vi "Launcher.vi"() -> ()   [LabVIEW 2024]
uses:
  <vilib>/Utility/miscctls.llb/LVRectTypeDef.ctl
  Factory Folder/EngineFactory/EngineFactory.lvclass
  Client Folder/Client/Client.lvclass
  Product Folder/IMotor/IMotor.lvclass
  Product Folder/IECU/IECU.lvclass
  <vilib>/addons/GOOPUtility/GOOPUtility.lvlib
panel:
  out "Error Out":errorcluster
  out "Throttle Result":string
  out "Degree Result":string
  in  "Apply Throttle":bool
  in  "Apply Degree":bool
  in  "Throttle":dbl min=0.0 max=100.0 format="%#_g %"
  in  "Degree":dbl
  out "ECU Type":string
  out "Motor Type":string
  in  "Create Engine Button":bool
  in  "Engine Type":string(combo)
  # "ENGINE TYPE"
  # "ECU TYPE"
  # "MOTOR TYPE"
  # "DEGREE"
  # "THROTTLE"
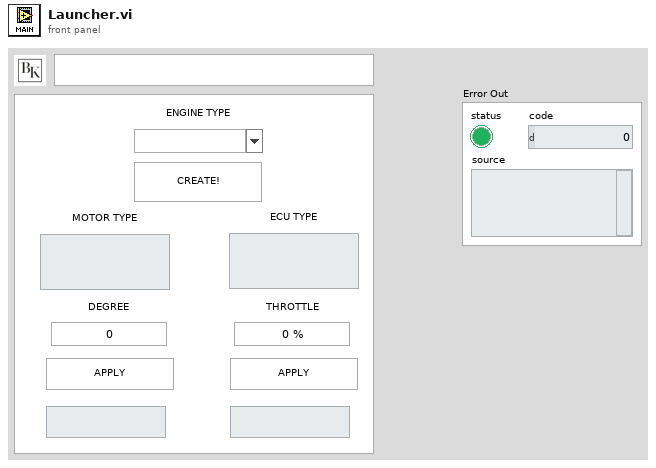
[diagram p1: front panel]
types:
  T1 = typedef "LVRectTypeDef.ctl" = cluster{"Left":i16, "Top":i16, "Right":i16, "Bottom":i16}
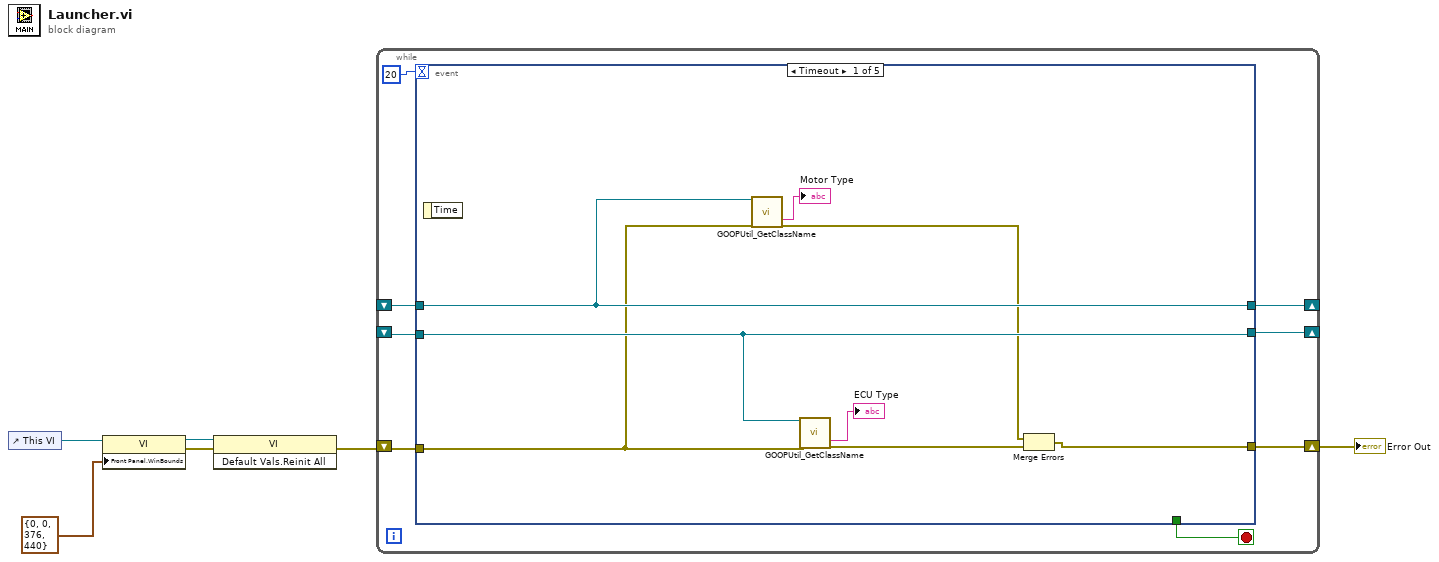
[diagram p0: block diagram]
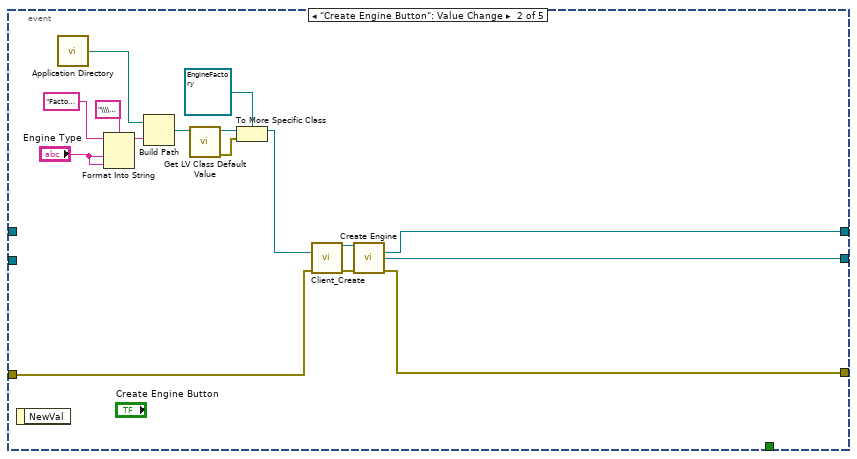
[diagram p2: hidden frame]
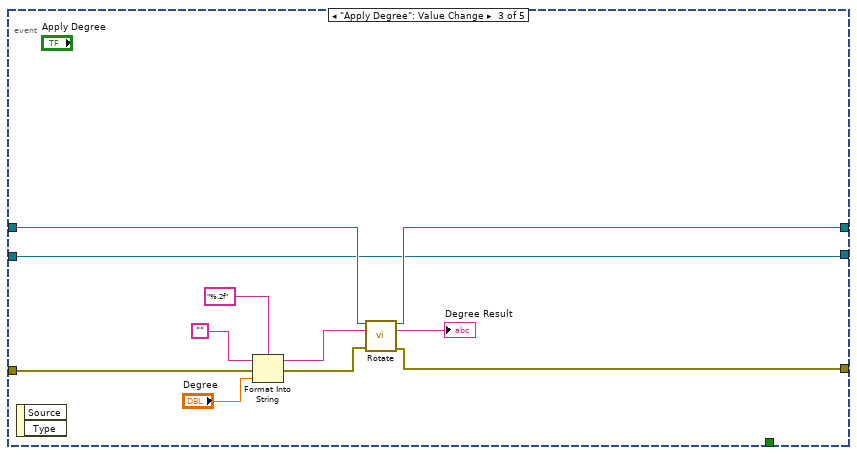
[diagram p3: hidden frame]
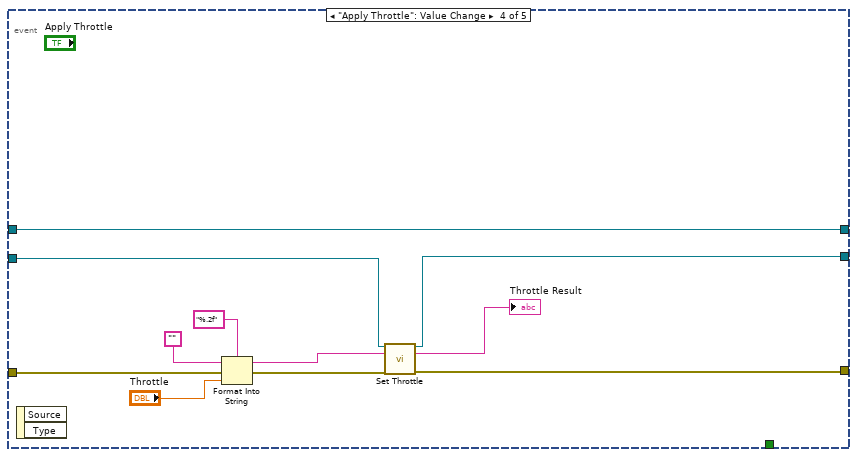
[diagram p4: hidden frame]
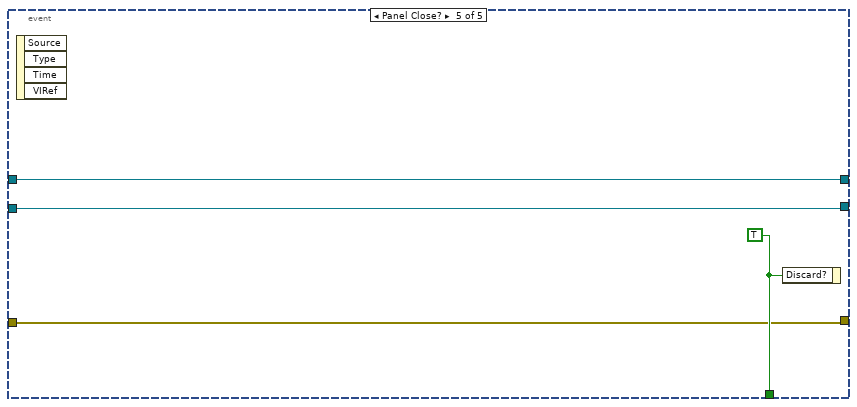
[diagram p5: hidden frame]
diagram:
  n1 = control-ref of="This VI"() -> (w4:refnum<vi>)
  n2 = property class="VI"(reference=w4, "Front Panel.WinBounds"=T1 {"Left"=0, "Top"=0, "Right"=376, "Bottom"=440} ("Front Panel Window:Window Bounds")) -> (reference out=w6:refnum<vi>, error out=w5:errorcluster)  [unwired: 1 in]
  n3 = invoke class="VI" method="Default Vals.Reinit All"(reference=w6, error in=w5) -> (error out=w2:errorcluster)  [unwired: 1 in, 2 out]
  n4 = while {
    shift-right: [w11] -> _
    shift-left: _ -> [w9]
    shift-right: [w10] -> _
    shift-left: _ -> [w8]
    shift-right: [w12] -> w1
    shift-left: w2 -> [w13]
    stop <- w14 stop-if-true
    n5 = event shown="[0] Timeout" {
      selector: _ -> [_ _ _ _ _]
      dyn-events: _ -> [_ _ _ _ _]
      timeout: 20 -> [_ _ _ _ _]
      tunnel: [_ _ _ _ w64] -> w14
      tunnel: w13 -> [w15 w38 w40 w51 w61]
      tunnel: [w17 w25 w45 w58 w61] -> w12
      tunnel: [w20 w24 w46 w53 w63] -> w11
      tunnel: [w19 w23 w42 w59 w62] -> w10
      tunnel: w9 -> [w20 _ w49 w53 w63]
      tunnel: w8 -> [w19 _ w42 w60 w62]
      event Timeout {
        n6 = event-data() -> ()  [unwired: 1 in, 1 out]
        n7 = call <vilib>:"GOOPUtil_GetClassName.vi"("LabVIEW Object"=w20, "error in (no error)"=w15) -> ("Full Class Name"=→"Motor Type":string, "error out"=w16:errorcluster)  [unwired: 13 in, 3 out]
        n8 = call <vilib>:"GOOPUtil_GetClassName.vi"("LabVIEW Object"=w19, "error in (no error)"=w15) -> ("Full Class Name"=→"ECU Type":string, "error out"=w22:errorcluster)  [unwired: 13 in, 3 out]
        n9 = Merge Errors(w16, w22) -> (w17:errorcluster)
      }
      event "Create Engine Button": Value Change {
        n10 = event-data() -> ()  [unwired: 1 in, 1 out]
        n11 = call <vilib>:"Application Directory.vi"() -> ("Application Directory"=w37:path)
        n12 = Format Into String(format string="\\\\%s\\\\%s.lvclass", initial string="Factory Folder" ("name or relative path"), "Engine Type", "Engine Type") -> (resulting string=w34:string)  [unwired: 1 in, 1 out]
        n13 = Build Path(base path=w37, name or relative path=w34) -> (appended path=w33:path)
        n14 = call <vilib>:"Get LV Class Default Value.vi"("class path"=w33) -> ("error out"=w29:errorcluster, "object"=w30:refnum<class>)  [unwired: 9 in]
        n15 = To More Specific Class(target class=refnum<class "EngineFactory.lvclass"> refnum ("EngineFactory"), reference=w30, error in=w29) -> (specific class reference=w28:refnum<class "EngineFactory.lvclass">)  [unwired: 1 out]
        n16 = call "Client_Create.vi"("Engine Factory"=w28, "Error In"=w38) -> ("reference out"=w27:refnum<class "Client.lvclass">, "Error Out"=w26:errorcluster)  [unwired: 12 in]
        n17 = call-dynamic "Create Engine.vi"("reference in"=w27, "Error In"=w26) -> ("Motor"=w24:refnum<class "IMotor.lvclass">, "ECU"=w23:refnum<class "IECU.lvclass">, "Error Out"=w25:errorcluster)  [unwired: 10 in, 1 out]
      }
      event "Apply Degree": Value Change {
        n18 = event-data() -> ()  [unwired: 1 in, 2 out]
        n19 = Format Into String(format string="%.2f", initial string="", error in=w40, "Degree") -> (resulting string=w48:string, error out=w39:errorcluster)
        n20 = call-dynamic "Rotate.vi"("object in"=w49, "Degree"=w48, "Error In"=w39) -> ("object out"=w46:refnum<class "IMotor.lvclass">, "Result"=→"Degree Result":string, "Error Out"=w45:errorcluster)  [unwired: 10 in]
      }
      event "Apply Throttle": Value Change {
        n21 = event-data() -> ()  [unwired: 1 in, 2 out]
        n22 = Format Into String(format string="%.2f", initial string="", error in=w51, "Throttle") -> (resulting string=w56:string, error out=w50:errorcluster)
        n23 = call-dynamic "Set Throttle.vi"("object in"=w60, "Throttle"=w56, "Error In"=w50) -> ("object out"=w59:refnum<class "IECU.lvclass">, "Result"=→"Throttle Result":string, "Error Out"=w58:errorcluster)  [unwired: 10 in]
      }
      event Panel Close? {
        w64 = TRUE ("Discard?")
        n24 = event-data() -> ()  [unwired: 1 in, 4 out]
        n25 = event-data("Discard?"=w64) -> ()  [unwired: 1 in, 1 out]
      }
    }
  }
  "Error Out" <- w1
